vi "McPherson Scan V1.00.vi"(3 "Point #":i32, 5 "Parameters":u8[](array[numeric])) -> (0 "Stop":bool, 1 "Data Out":dbl[](array[numeric]) format="%.2f")   [LabVIEW 2020]
uses:
  Globals and TypeDefs/Global Varibal Control.vi
panel:
  out "vi state":enum32{"Broken", "Idle", "Running"}(ring)
  out "window state":enum32{"Closed", "Open", "Open and Active"}(ring)
  out "Position":dbl format="%.2f"
  # "Scanning Pattern"
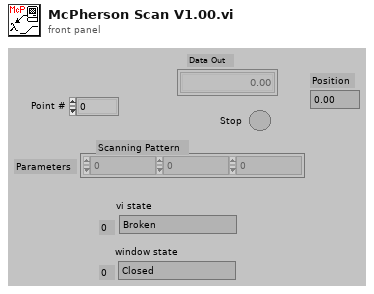
[diagram p1: front panel]
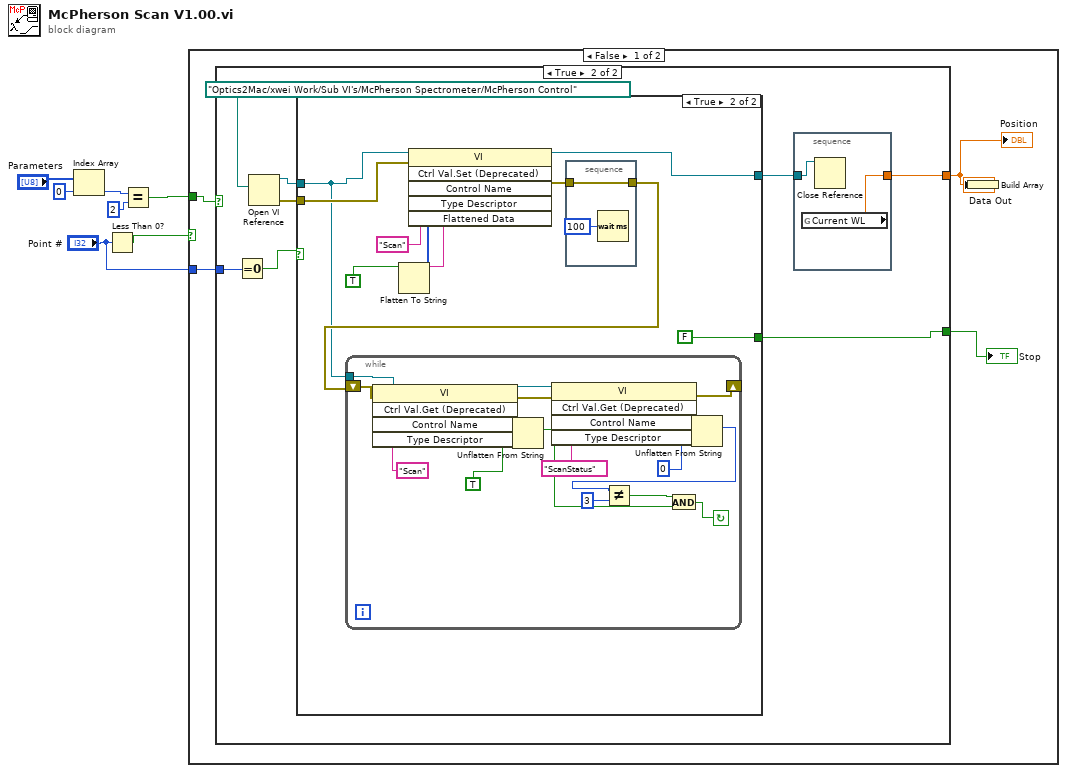
[diagram p0: block diagram]
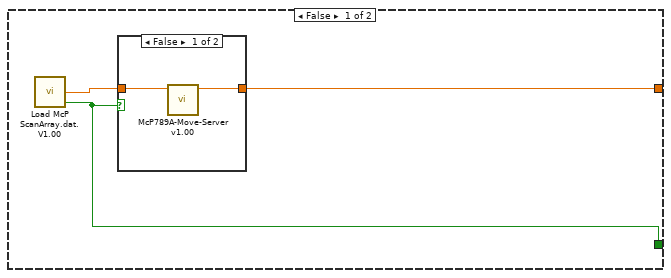
[diagram p2: hidden frame]
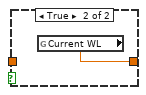
[diagram p3: hidden frame]
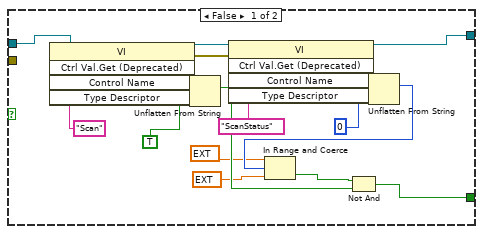
[diagram p4: hidden frame]
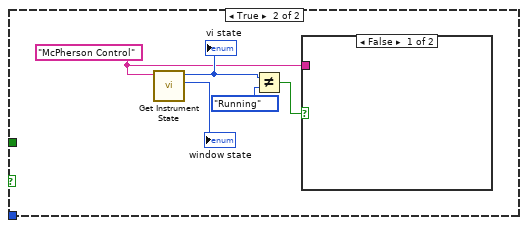
[diagram p5: hidden frame]
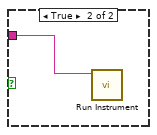
[diagram p6: hidden frame]
diagram:
  n1 = Index Array(array="Parameters", index=0 ("Index")) -> (element=w4:u8)
  n2 = Less Than 0?(x="Point #") -> (x < 0?=w7:bool)
  n3 = Equal?(x=w4, y=u8 2) -> (x = y?=w2:bool)
  n4 = case shown="False" w7 {
    tunnel: w2 -> [w9 _]
    tunnel: "Point #" -> [w8 _]
    frame False {
      n5 = case shown="True" w9 {
        tunnel: [w14 w26] -> w12
        tunnel: [w13 w19] -> w10
        tunnel: w8 -> [_ w25]
        frame False {
          n6 = call "Load McP ScanArray.dat.V1.00.vi"() -> ("Position"=w15:sgl, "EOF?"=w14:bool)  [unwired: 2 in, 1 out]
          n7 = case shown="False" w14 {
            tunnel: w15 -> [w17 _]
            tunnel: [w16 w18] -> w13
            frame False {
              n8 = call "McP789A-Move-Server v1.00.vi"("GOTO"=w17) -> ("CurrentPosition"=w16:dbl)  [unwired: 7 in, 2 out]
            }
            frame True {
              n9 = global read "Global Varibal Control.vi" "Current WL"() -> (w18:dbl)
            }
          }
        }
        frame True {
          n10 = Equal To 0?(x=w25) -> (x = 0?=w24:bool)
          n11 = Open VI Reference(vi path=path "/Optics2Mac/xwei Work/Sub VI's/McPherson Spectrometer/McPherson Control") -> (vi reference=w22:refnum<vi>, error out=w23:errorcluster)  [unwired: 5 in]
          n12 = case shown="True" w24 {
            tunnel: w22 -> [w34 w45]
            tunnel: [w35 FALSE] -> w26
            tunnel: w23 -> [_ w54]
            tunnel: [w29 w47] -> w20
            frame False {
              n13 = invoke class="VI" method="Ctrl Val.Get (Deprecated)"(reference=w34, "Control Name"="Scan") -> (reference out=w39:refnum<vi>, error out=w38:errorcluster, "Get Control Value"=w40:string)  [unwired: 3 in, 2 out]
              n14 = Unflatten From String(type=TRUE ("Wait until done"), binary string=w40) -> (value=w36:bool)  [unwired: 3 in, 2 out]
              n15 = invoke class="VI" method="Ctrl Val.Get (Deprecated)"(reference=w39, error in=w38, "Control Name"="ScanStatus") -> (reference out=w29:refnum<vi>, "Get Control Value"=w43:string)  [unwired: 2 in, 3 out]
              n16 = Unflatten From String(type=u8 0, binary string=w43) -> (value=w33:u8)  [unwired: 3 in, 2 out]
              n17 = In Range and Coerce(upper limit=ext 4.1 ("hi"), x=w33, lower limit=ext 2.9 ("lo")) -> (In Range?=w32:bool)  [unwired: 1 out]
              n18 = Not And(1:w36, 2:w32) -> (0:w35:bool)
            }
            frame True {
              n19 = Flatten To String(anything=TRUE ("Wait until done")) -> (data string=w49:string, type string=w52:i16[])  [unwired: 3 in, 1 out]
              n20 = invoke class="VI" method="Ctrl Val.Set (Deprecated)"(reference=w45, error in=w54, "Control Name"="Scan", "Type Descriptor"=w52, "Flattened Data"=w49) -> (reference out=w47:refnum<vi>, error out=w53:errorcluster)  [unwired: 1 in, 4 out]
              n21 = stacked-sequence {
                tunnel: [w71] -> w46
                tunnel: w53 -> [w71]
                frame #0 {
                  n22 = Wait (ms)(milliseconds to wait=u32 100) -> ()  [unwired: 1 out]
                }
              }
              n23 = while {
                tunnel: w45 -> [w57]
                shift-left: w46 -> [w59]
                shift-right: [w58] -> _
                stop <- w68 continue-if-true
                n24 = invoke class="VI" method="Ctrl Val.Get (Deprecated)"(reference=w57, error in=w59, "Control Name"="Scan") -> (reference out=w62:refnum<vi>, error out=w61:errorcluster, "Get Control Value"=w63:string)  [unwired: 2 in, 2 out]
                n25 = Unflatten From String(type=TRUE ("Wait until done"), binary string=w63) -> (value=w55:bool)  [unwired: 3 in, 2 out]
                n26 = invoke class="VI" method="Ctrl Val.Get (Deprecated)"(reference=w62, error in=w61, "Control Name"="ScanStatus") -> (error out=w58:errorcluster, "Get Control Value"=w66:string)  [unwired: 2 in, 3 out]
                n27 = Unflatten From String(type=u8 0, binary string=w66) -> (value=w56:u8)  [unwired: 3 in, 2 out]
                n28 = Not Equal?(x=w56, y=u8 3) -> (x != y?=w69:bool)
                n29 = And(x=w69, y=w55) -> (x .and. y?=w68:bool)
              }
            }
          }
          n30 = stacked-sequence {
            tunnel: w20 -> [w28]
            tunnel: [w27] -> w19
            frame #0 {
              n31 = global read "Global Varibal Control.vi" "Current WL"() -> (w27:dbl)
              n32 = Close Reference(reference=w28) -> ()  [unwired: 1 in, 1 out]
            }
          }
        }
      }
      "Stop" <- w12
      "Position" <- w10
      n33 = Build Array(w10) -> (→"Data Out":dbl[])
    }
    frame True {
      w73 = "McPherson Control" ("VI name")
      n34 = call <vilib>:"Get Instrument State.vi"("VI name"=w73) -> ("window state"=→"window state":enum32{"Closed", "Open", "Open and Active"}, "vi state"=w76:enum32{"Broken", "Idle", "Running"})  [unwired: 8 in, 1 out]
      "vi state" <- w76
      n35 = Not Equal?(x=w76, y=enum32{"Broken", "Idle", "Running"}."Running") -> (x != y?=w74:bool)
      n36 = case shown="False" w74 {
        tunnel: w73 -> [_ w78]
        frame False {
        }
        frame True {
          n37 = call <vilib>:"Run Instrument.vi"("VI name"=w78) -> ()  [unwired: 10 in, 1 out]
        }
      }
    }
  }
